vi "Servo Motor.vi"(8 "Error In":errorcluster, 9 "Position":i32, 10 "Servo Channel":u8=6, 11 "LINX Resource In":T1) -> (0 "Error Out":errorcluster, 2 "Angle":u16, 3 "LINX Resource Out":T1)   [LabVIEW 2020]
uses:
  <vilib>/MakerHub/LINX/Private/Type Defs/LINX Ref.ctl
  <vilib>/MakerHub/LINX/Private/Type Defs/Platform.ctl
  <vilib>/MakerHub/LINX/Private/Type Defs/Interface.ctl
  <vilib>/MakerHub/LINX/Private/Device/Type Defs/LINX Device Config.ctl
  <vilib>/MakerHub/LINX/Private/Device/Type Defs/TCP Config.ctl
  <vilib>/MakerHub/LINX/Private/Device/Type Defs/Channels.ctl
  <vilib>/MakerHub/LINX/Public/Sensors/Motion/Servo/Servo Set Pulse Width One Channel.vi
  <vilib>/MakerHub/LINX/Public/Sensors/Motion/Servo/Servo.lvlib
  <vilib>/Analysis/NI_AALPro.lvlib
  <vilib>/MakerHub/LINX/LMH-LINX.lvlib
  <vilib>/MakerHub/LINX/Private/Device/Device.lvlib
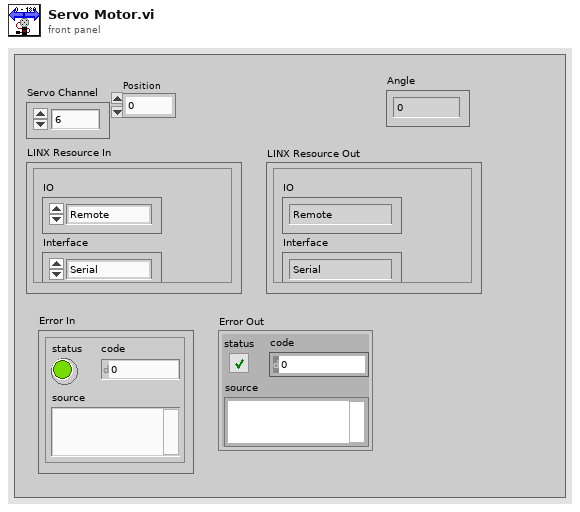
[diagram p1: front panel]
types:
  T1 = typedef "LMH-LINX.lvlib/LINX Ref.ctl" = cluster{"IO":T2, "Interface":T3, "LINX Device Config":T4}
  T2 = typedef "LMH-LINX.lvlib/Platform.ctl" = enum16{"Remote", "Local"}
  T3 = typedef "LMH-LINX.lvlib/Interface.ctl" = enum16{"Serial", "TCP"}
  T4 = typedef "LMH-LINX.lvlib/Device.lvlib/LINX Device Config.ctl" = cluster{"Interface":T3, "COM Port":refnum<visa-resource-name>, "TCP Configuration":T5, "Device Family":u8, "Device ID":u8, "Device Name":string, "TCP Ref":refnum<k5>, "Channels":T6}
  T5 = typedef "LMH-LINX.lvlib/Device.lvlib/TCP Config.ctl" = cluster{"IP Address":string, "Port":u16}
  T6 = typedef "LMH-LINX.lvlib/Channels.ctl" = cluster{"DI":u8[], "DO":u8[], "AI":u8[], "AO":u8[], "PWM":u8[], "QE":u8[], "UART":u8[], "I2C 2":u8[], "SPI":u8[], "CAN":u8[], "Servo":u8[], "AI Ref (V)":dbl, "AI Resolution (Bits)":u8, "AO Ref (V)":dbl, "AO Resolution (Bits)":u8}
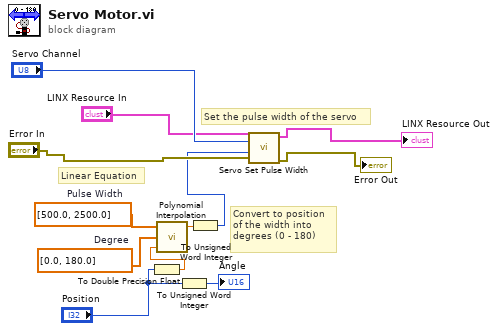
[diagram p0: block diagram]
diagram:
  w6 = dbl[] [0.0, 180.0]  # Degree
  w7 = dbl[] [500.0, 2500.0]  # Pulse Width
  # "Linear Equation"
  # "Set the pulse width of the servo"
  # "Convert to position\nof the width into \ndegrees (0 - 180)"
  n1 = To Double Precision Float(number="Position") -> (double precision float=w2:dbl)
  n2 = call <vilib>:"Polynomial Interpolation.vi"("x value"=w2, "X"=w6, "Y"=w7) -> ("interpolation value"=w5:dbl)  [unwired: 2 out]
  n3 = To Unsigned Word Integer(number="Position") -> (unsigned 16bit integer=→"Angle":u16)
  n4 = To Unsigned Word Integer(number=w5) -> (unsigned 16bit integer=w4:u16)
  n5 = call-poly <vilib>:"Servo Set Pulse Width.vi"("Error In"="Error In", "Pulse Width (uS)"=w4, "Servo Channel"="Servo Channel", "LINX Resource"="LINX Resource In") -> ("Error Out"=→"Error Out":errorcluster, "LINX Resource"=→"LINX Resource Out":T1)  [unwired: 6 in]
